vi "html_extract_form.vi"(11 "Message Body":string) -> (3 "Form Data":T1[](array[typedef]))   [LabVIEW 2011]
uses:
  html_form_field.ctl
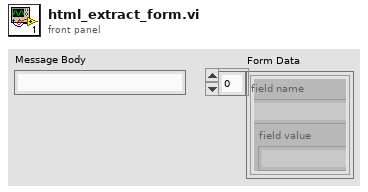
[diagram p1: front panel]
types:
  T1 = typedef "html_form_field.ctl" = cluster{"field name":string, "field value":string}
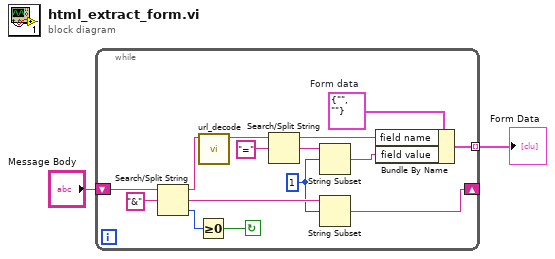
[diagram p0: block diagram]
diagram:
  n1 = while {
    shift-right: [w14] -> _
    shift-left: "Message Body" -> [w17]
    tunnel: [w12] -> w1 mode=indexing
    stop <- w9 continue-if-true
    w3 = u8 1 ("default (0 U32)")
    w13 = T1 {"field name"="", "field value"=""}  # Form data
    n2 = Search/Split String(string=w17, search string/char (-)="&") -> (substring before match=w11:string, match + rest of string=w16:string, offset of match=w10:i32)  [unwired: 1 in]
    n3 = Greater Or Equal To 0?(x=w10) -> (x >= 0?=w9:bool)
    n4 = call "url_decode.vi"("Message Body in"=w11) -> ("Message Body out"=w8:string)  [unwired: 10 in]
    n5 = Search/Split String(string=w8, search string/char (-)="=") -> (substring before match=w6:string, match + rest of string=w5:string)  [unwired: 1 in, 1 out]
    n6 = String Subset(string=w5, offset (0)=w3) -> (substring=w4:string)  [unwired: 1 in]
    n7 = String Subset(string=w16, offset (0)=w3) -> (substring=w14:string)  [unwired: 1 in]
    n8 = Bundle By Name(cluster=w13, "field name"=w6, "field value"=w4) -> (w12:T1)
  }
  "Form Data" <- w1
